vi "Script Read HW Types Accessor Value.vi"(8 "error in (no error)":errorcluster, 10 "Project in":refnum<vi>, 11 "MeasurementMetaData in":refnum<class "MeasurementMetaData.lvclass">) -> (0 "error out":errorcluster, 3 "MeasurementMetaData out":refnum<class "MeasurementMetaData.lvclass">)   [LabVIEW 2013, in "MeasurementMetaData.lvclass"]
doc: "This code modifies the method that returns the required hardware types based upon what the user selected in the configuration dialog."
uses:
  MeasurementMetaData.lvclass
  MeasurementMetaData.lvclass/MeasurementMetaData.ctl
  <resource>/dialog/NewProjectWizard/MetaDataObj/MetaDataObj.lvclass
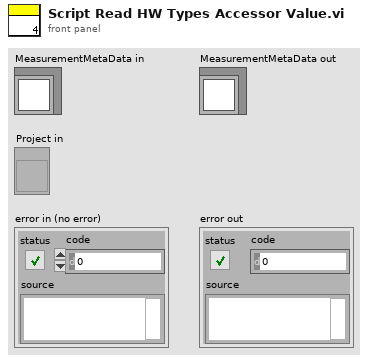
[diagram p1: front panel]
types:
  T1 = typedef "MeasurementMetaData.lvclass/Plugin Settings.ctl" = cluster{"Override Configure Method":bool, "Generate Custom Results Object":bool, "Override Measure Method":bool, "Override Close Method":bool, "Scope?":bool, "DMM?":bool, "FGEN?":bool, "PSU?":bool, "Acquisition Mode":enum16{"Continuous", "Single-Shot"}}
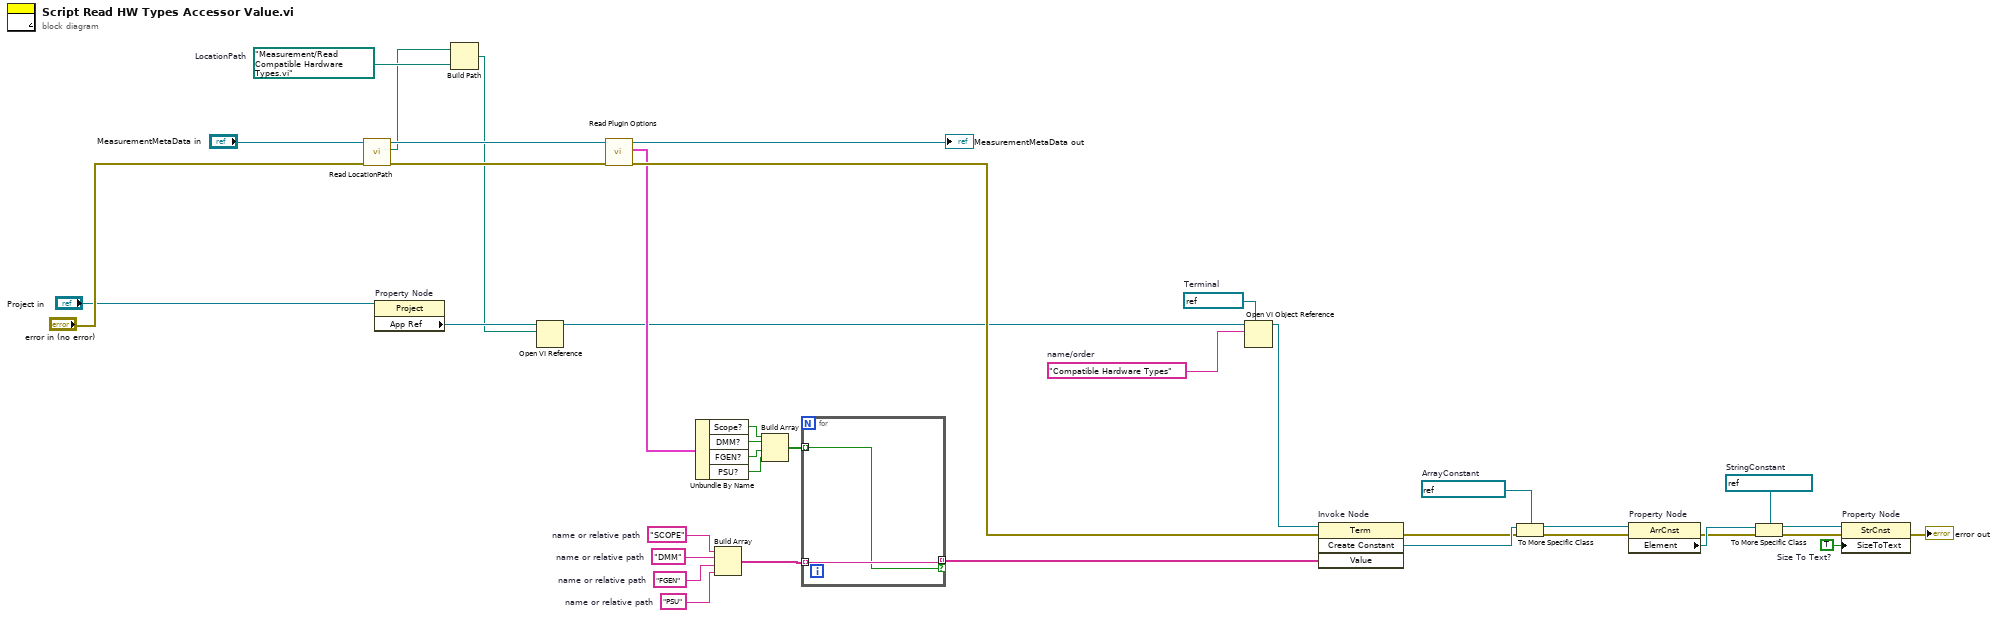
[diagram p0: block diagram]
diagram:
  w39 = TRUE  # Size To Text?
  w36 = refnum<vi> refnum  # StringConstant
  w31 = refnum<vi> refnum  # ArrayConstant
  w20 = refnum<vi> refnum  # Terminal
  w19 = "Compatible Hardware Types"  # name/order
  w10 = "PSU"  # name or relative path
  w13 = "SCOPE"  # name or relative path
  w11 = "FGEN"  # name or relative path
  w12 = "DMM"  # name or relative path
  w2 = path "Measurement/Read Compatible Hardware Types.vi"  # LocationPath
  n1 = call <resource>:"Read LocationPath.vi"("error in (no error)"="error in (no error)", "MetaDataObj in"="MeasurementMetaData in") -> ("error out"=w9:errorcluster, "LocationPath"=w1:path, "MetaDataObj out"=w7:refnum<class "MeasurementMetaData.lvclass">)  [unwired: 7 in]
  n2 = property on="Property Node" class="Project"(reference="Project in") -> ("App Ref"=w17:refnum<vi>)  [unwired: 1 in, 2 out]
  n3 = Build Path(base path=w1, name or relative path=w2) -> (appended path=w3:path)
  n4 = Open VI Reference(application reference (local)=w17, vi path=w3) -> (vi reference=w18:refnum<vi>)  [unwired: 4 in, 1 out]
  n5 = call "Read Plugin Options.vi"("error in (no error)"=w9, "MeasurementMetaData in"=w7) -> ("error out"=w24:errorcluster, "Plugin Options"=w22:T1, "MeasurementMetaData out"=→"MeasurementMetaData out":refnum<class "MeasurementMetaData.lvclass">)  [unwired: 7 in]
  n6 = Unbundle By Name "Unbundle By Name"(w22) -> ("Scope?"=w28:bool, "DMM?"=w16:bool, "FGEN?"=w15:bool, "PSU?"=w14:bool)
  n7 = Build Array "Build Array"(w13, w12, w11, w10) -> (w26:string[])
  n8 = Build Array(w28, w16, w15, w14) -> (w23:bool[])
  n9 = for {
    tunnel: w23 -> [w40] mode=indexing
    tunnel: w26 -> [w41] mode=indexing
    tunnel: [w41] -> w27 mode=indexing if=w40
  }
  n10 = Open VI Object Reference(7:w20, 10:w19, 11:w18) -> (3:w21:refnum<vi>)  [unwired: 1 in, 1 out]
  n11 = invoke on="Invoke Node" class="Term" method="Create Constant"(reference=w21, error in=w24, "Value"=w27) -> (error out=w25:errorcluster, "Create Constant"=w30:refnum<vi>)  [unwired: 1 in, 2 out]
  n12 = To More Specific Class(target class=w31, reference=w30, error in=w25) -> (specific class reference=w33:refnum<vi>, error out=w29:errorcluster)
  n13 = property on="Property Node" class="ArrCnst"(reference=w33, error in=w29) -> (error out=w32:errorcluster, "Element"=w35:refnum<vi>)  [unwired: 1 out]
  n14 = To More Specific Class(target class=w36, reference=w35, error in=w32) -> (specific class reference=w38:refnum<vi>, error out=w34:errorcluster)
  n15 = property on="Property Node" class="StrCnst"(reference=w38, error in=w34, "SizeToText"=w39) -> (error out=→"error out":errorcluster)  [unwired: 1 out]
